vi "Find VI Ref.vi"(8 "error in":errorcluster, 9 "VI Name":string, 10 "Owned Items[]":refnum<vi>[](array[refnum])) -> (0 "error out":errorcluster, 1 "VI Ref":refnum<vi>)   [LabVIEW 2025, in "_Rename.lvlib" / "_Rename.lvclass"]
uses:
  _Rename.lvclass
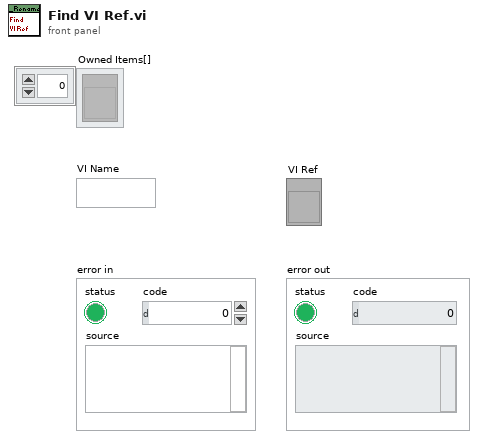
[diagram p1: front panel]
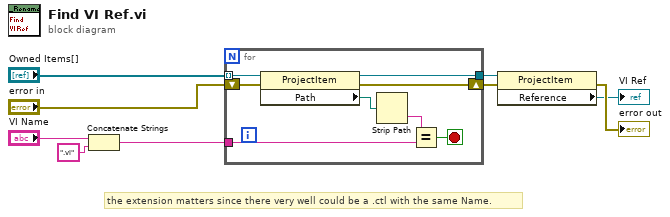
[diagram p0: block diagram]
diagram:
  # "the extension matters since there very well could be a .ctl with the same Name."
  # "the extension matters since there very well could be a .ctl with the same Name."
  n1 = Concatenate Strings("VI Name", ".vi" ("string")) -> (w2:string)
  n2 = for {
    tunnel: "Owned Items[]" -> [w17] mode=indexing
    shift-right: [w15] -> w8
    shift-left: "error in" -> [w16]
    tunnel: [w14] -> w9
    tunnel: w2 -> [w10]
    stop <- w13 stop-if-true
    n3 = property class="ProjectItem"(reference=w17, error in=w16) -> (reference out=w14:refnum<vi>, error out=w15:errorcluster, "Path"=w12:path)
    n4 = Strip Path(path=w12) -> (name=w11:string)  [unwired: 1 out]
    n5 = Equal?(x=w11, y=w10) -> (x = y?=w13:bool)
  }
  n6 = property class="ProjectItem"(reference=w9, error in=w8) -> (error out=→"error out":errorcluster, "Reference"=→"VI Ref":refnum<vi>)  [unwired: 1 out]
